vi "Billard2025.vi"(5 "Open pdf":bool=TRUE, 7 "ball size":i32=13, 8 "band touch win":u32(colorbox)=16711680, 9 "band touch loose":u32(colorbox)=6618880, 10 "Open Scoresheet":bool=TRUE, 11 "path to PNG file":path=path "/Users/leonkesselring/Desktop/LabView/Proj Prog/T1-2") -> (0 "error out":errorcluster={"status"=TRUE, "code"=-1, "source"="Script error. \n{\bError: File: /Users/leonkesselring/Desktop/LabView/Proj Prog/AnalyseT5.m Line:\n310 Column: 34\nThe function \"GetTouchIdx\" was closed with an 'end', but at least one other\nfunction definition was not. All functions in a script must be closed with an\n'end'.\n}\b \n"}, 1 "Summary output":string="Error -1 occurred at Script error. \n{\bError: File: /Users/leonkesselring/Desktop/LabView/Proj Prog/AnalyseT5.m Line:\n310 Column: 34\nThe function \"GetTouchIdx\" was closed with an 'end', but at least one other\nfunction definition was not. All functions in a script must be closed with an\n'end'.\n}\b\n\nThis error code is undefined. Undefined errors might occur for a number of reasons. For example, no one has provided a description for the code, or you might have wired a number that is not an error code to the error code input. \n\nAdditionally, undefined error codes might occur because the error relates to a third-party object, such as the operating system or ActiveX. For these third-party errors, you might be able to obtain a description of the error by searching the Web for the error code (-1) or for its hexadecimal representation (0xFFFFFFFF).")   [LabVIEW 2025]
panel:
  out "error out 3":errorcluster={"status"=TRUE, "code"=-1, "source"="Script error. \n{\bError: File: /Users/leonkesselring/Desktop/LabView/Proj Prog/AnalyseT5.m Line:\n310 Column: 34\nThe function \"GetTouchIdx\" was closed with an 'end', but at least one other\nfunction definition was not. All functions in a script must be closed with an\n'end'.\n}\b \n"}
  out "error out 2":errorcluster
  out "stripped path txt file 3":path=path "/Users/leonkesselring/Desktop/LabView/Proj Prog"
  out "name":string="T5"
  out "filenames":string[](array[string])=["1591.png", "1592.png", "1593.png", "1594.png", "1595.png", "1596.png", "1597.png", "1598.png", "1599.png", "1600.png", "1601.png", "1602.png", "1603.png", "1604.png", "1605.png", "1606.png", "1607.png", "1608.png", "1609.png", "1610.png", "1611.png", "1612.png", "1613.png", "1614.png", "1615.png", "1616.png", "1617.png", "1618.png", "1619.png", "1620.png", "1621.png", "1622.png", "1623.png", "1624.png", "1625.png", "1626.png", "1627.png", "1628.png", "1629.png", "1630.png", "1631.png", "1632.png", "1633.png", "1634.png", "1635.png", "1636.png", "1637.png", "1638.png", "1639.png", "1640.png", "1641.png", "1642.png", "1643.png", "1644.png", "1645.png", "1646.png", "1647.png", "1648.png", "1649.png", "1650.png", "1651.png", "1652.png", "1653.png", "1654.png", "1655.png", "1656.png", "1657.png", "1658.png", "1659.png", "1660.png", "1661.png", "1662.png", "1663.png", "1664.png", "1665.png", "1666.png", "1667.png", "1668.png", "1669.png", "1670.png", "1671.png", "1672.png", "1673.png", "1674.png", "1675.png", "1676.png", "1677.png", "1678.png", "1679.png", "1680.png", "1681.png", "1682.png", "1683.png", "1684.png", "1685.png", "1686.png", "1687.png", "1688.png", "1689.png", "1690.png", "1691.png", "1692.png", "1693.png", "1694.png", "1695.png", "1696.png", "1697.png", "1698.png", "1699.png", "1700.png", "1701.png", "1702.png", "1703.png", "1704.png", "1705.png", "1706.png", "1707.png", "1708.png", "1709.png", "1710.png", "1711.png", "1712.png", "1713.png", "1714.png", "1715.png", "1716.png", "1717.png", "1718.png", "1719.png", "1720.png", "1721.png", "1722.png", "1723.png", "1724.png", "1725.png", "1726.png", "1727.png", "1728.png", "1729.png", "1730.png", "1731.png", "1732.png"]
  out "String":string="T5"
  out "concatenated string":string="\n \nTlist;%% integrating \"InterpolateNan\" and \"RemoveOutlier\"\n\n% Interpolate missing values in the traces\n[Xr, Yr] = InterpolateNan(Xr, Yr);\n[Xy, Yy] = InterpolateNan(Xy, Yy);\n[Xw, Yw] = InterpolateNan(Xw, Yw);\n\n% Remove outliers from the traces\n[Xr, Yr] = RemoveOutlier(Xr, Yr);\n[Xy, Yy] = RemoveOutlier(Xy, Yy);\n[Xw, Yw] = RemoveOutlier(Xw, Yw);\n\n%% invert\nH = 480;\nYr = H - Yr;\nYy = H - Yy;\nYw = H - Yw;\n\n%% integrating \"GetFramme\"\n\n[Xmin, Xmax, Ymin, Ymax] = GetFrame(Xr, Yr, Xy, Yy, Xw, Yw);\n\n\n%% creat trace for frame\n\nxf = [Xmin Xmax Xmax Xmin Xmin];\nyf = [Ymin Ymin Ymax Ymax Ymin];\n\n%% integrating \"GetBallPathLength\" and \"GetFirstMoveIdx\"\nMoveDistPx = 9;\nLr = GetBallPathLength(Xr, Yr);\nLy = GetBallPathLength(Xy, Yy);\nLw = GetBallPathLength(Xw, Yw);\n\n[idxFirstR, DistMoveR] = GetFirstMoveIdx(Xr, Yr, MoveDistPx);\n[idxFirstY, DistMoveY] = GetFirstMoveIdx(Xy, Yy, MoveDistPx);\n[idxFirstW, DistMoveW] = GetFirstMoveIdx(Xw, Yw, MoveDistPx);\n\n%% integrating \"GetTouchIdx\" and \"GetBallMoveOrder\"\n\nBallBorderDist = 9;\nIdxTouchR = GetTouchIdx(Xr, Yr, Xmin, Xmax, Ymin, Ymax, BallBorderDist);\nIdxTouchY = GetTouchIdx(Xy, Yy, Xmin, Xmax, Ymin, Ymax, BallBorderDist);\nIdxTouchW = GetTouchIdx(Xw, Yw, Xmin, Xmax, Ymin, Ymax, BallBorderDist);\n\n[FirstBall, SecondBall, LastBall, NbBallsMoved] = GetBallMoveOrder(Xr, Yr, Xy, Yy, Xw, Yw, MoveDistPx);\n\nif FirstBall == 1\n    Xfirst = Xr;\n    Yfirst = Yr;\n    IdxTouchfirst = IdxTouchR;\n    ColorScore = 'red';\nelseif FirstBall == 2\n    Xfirst = Xy;\n    Yfirst = Yy;\n    IdxTouchfirst = IdxTouchY;\n    ColorScore = 'yellow';\nelse \n    Xfirst = Xw;\n    Yfirst = Yw;\n    IdxTouchfirst = IdxTouchW;\n    ColorScore = 'white';\nend\n\n%% determin Win/lose\n\nScore = GetWinnerScore(idxFirstR, idxFirstY, idxFirstW, IdxTouchfirst, NbBallsMoved);\n\nif strcmp(Score, 'win')\n    \n\ncolortouches = [1 0 0];\nelse\ncolortouches = [0 1 0];\nend\n%% Display the frame and traces\n\nfig = figure('Color','k'); % dark background\nax = axes(fig);\nset(ax,'Color','k'); \nhold(ax,'on'); \n\n% Frame in gray\nplot(ax, xf, yf, '-', 'LineWidth', 1.5, 'Color', [0.6 0.6 0.6]);\n\n% Traces: R, Y, W\nplot(ax, Xr, Yr, 'o-', 'LineWidth', 1.6, 'Color', [1 0 0]);   % red\nplot(ax, Xy, Yy, 'o-', 'LineWidth', 1.6, 'Color', [1 1 0]);   % yellow\nplot(ax, Xw, Yw, 'o-', 'LineWidth', 1.6, 'Color', 'b');       % white ball (blue trace)\n\n% Plot touches for first ball\nplot(ax, Xfirst(IdxTouchfirst), Yfirst(IdxTouchfirst), 'o', ...\n     'MarkerSize', 30, 'Color', colortouches);\n\n% Plot origins\nplot(ax, Xr(1), Yr(1), 'hexagram', 'MarkerSize', 20, 'Color', [1 0 0]);\nplot(ax, Xy(1), Yy(1), 'hexagram', 'MarkerSize', 20, 'Color', [1 1 0]);\nplot(ax, Xw(1), Yw(1), 'hexagram', 'MarkerSize', 20, 'Color', 'b');\n\n% Design: frame sizing\naxis(ax,'equal');\naxis(ax,[Xmin Xmax Ymin Ymax]);\n\naxis(ax,'off');   \n\ntitle(ax, ['Scores sheet -T5 - ' datestr(now,'yyyy-mm-dd - HH:MM')], ...\n    'Color', 'w', 'FontSize', 14);\n\n\n%% Legend area below the frame\n\npadBottom = 0.20*(Ymax - Ymin);   \naxis(ax,[Xmin Xmax Ymin - padBottom Ymax]);\n\nxl = xlim(ax);\nyl = ylim(ax);\n\nxLeft   = xl(1) + 0.05*(xl(2)-xl(1));\nxCenter = xl(1) + 0.40*(xl(2)-xl(1));\nxRight  = xl(1) + 0.80*(xl(2)-xl(1));\nyBase   = yl(1) + 0.15*(Ymax - Ymin);\n\nNbBandsTouched = numel(IdxTouchfirst);\n\n% Winner section\nV = [idxFirstR idxFirstY idxFirstW];\nVsort = sort(V);\n\nif NbBallsMoved == 3   % only then Vsort has 3 elements\n    count = IdxTouchfirst( (Vsort(2) < IdxTouchfirst) & (IdxTouchfirst < Vsort(3)) );\n    NbBandsWin = numel(count);\nelse\n    NbBandsWin = 0;\nend\n\nif NbBallsMoved == 3 && NbBandsWin >= 3\n    Score = 'win';\nelse\n    Score = 'lose';\nend\n\n\ntext(xLeft, yBase, sprintf('Score sheet for \"%s\"', ColorScore), 'Color', 'w', 'FontSize', 12);\ntext(xLeft, yBase-30, sprintf('--- %s ---', Score), 'Color', 'w', 'FontSize', 12);\n\n% Distances\ntext(xLeft,   yBase-80, sprintf('red_d : %.0fpx',   Lr), 'Color', 'w', 'FontSize', 12);\ntext(xCenter, yBase-80, sprintf('yellow_d : %.0fpx', Ly), 'Color', 'w', 'FontSize', 12);\ntext(xRight,  yBase-80, sprintf('white_d : %.0fpx', Lw), 'Color', 'w', 'FontSize', 12);\n\n% Ball & band stats\ntext(xRight, yBase,   sprintf('%d ball(s) moved',   NbBallsMoved),   'Color', 'w', 'FontSize', 12);\ntext(xRight, yBase-30, sprintf('%d band(s) touched', NbBandsTouched), 'Color', 'w', 'FontSize', 12);\n\n%% PDF\nSeqName = 'T5';   % or pass this as a variable instead of hardcoding\r\n\r\npdfName = sprintf('ScoreSheet%s.pdf', SeqName);\r\nexportgraphics(fig, pdfName, 'ContentType','vector');\r\n\r\n%% Summary\r\n\r\n% Map ColorScore to char: f:[w,y,r]\r\nswitch lower(ColorScore)\r\n    case 'white'\r\n        fChar = 'w';\r\n    case 'yellow'\r\n        fChar = 'y';\r\n    case 'red'\r\n        fChar = 'r';\r\n    otherwise\r\n        fChar = 'x';   % unknown, for safety\r\nend\r\n\r\n% Map Score 'win'/'lose' to s:[w,l]\r\nif strcmpi(Score, 'win')\r\n    sChar = 'w';\r\nelse\r\n    sChar = 'l';\r\nend\r\n\r\n% Round distances to integers\r\nrb = round(Lr);\r\nyb = round(Ly);\r\nwb = round(Lw);\r\n\r\nsummaryStr = sprintf('f:%c; s:%c; n:%d; b:%d; rb:%d; yb:%d; wb:%d;', ...\r\n    fChar, sChar, NbBallsMoved, NbBandsTouched, rb, yb, wb);\r\n\r\nSummaryName = sprintf('Summary%s.txt', SeqName);\r\n\r\nfid = fopen(SummaryName, 'w');\r\nfprintf(fid, '%s\\n', summaryStr);\r\nfclose(fid);\r\n\r\n%% function InterpolateNan\r\n\r\nfunction [X, Y] = InterpolateNan(X, Y)\r\n\r\n    if isnan(X(1)),  X(1)  = 0; end\r\n    if isnan(X(end)),X(end)= 0; end\r\n\r\n    defX = ~isnan(X);\r\n    idX = 1:numel(X);\r\n    idx_defX = find(defX);\r\n    X =interp1(idx_defX,X(defX),idX,'next');\r\n\r\n    if isnan(Y(1)),  Y(1)  = 0; end\r\n    if isnan(Y(end)),Y(end)= 0; end\r\n\r\n    defY = ~isnan(Y);\r\n    idY = 1:numel(Y);\r\n    idx_defY = find(defY);\r\n    Y =interp1(idx_defY,Y(defY),idY,'next');\r\nend\r\n%% function RemoveOutlier\r\n\r\nfunction [X, Y] = RemoveOutlier(X, Y)\r\n    OX =isoutlier(X,'movmedian',10);\r\n    OY =isoutlier(Y,'movmedian',10);\r\n\r\n    O = OX & OY;\r\n    idx = find(O);\r\n    idx = idx(idx > 1);\r\n    \r\n    X(idx) = X(idx - 1);\r\n    Y(idx) = Y(idx - 1);\r\nend\r\n\r\n%% function GetFrame\r\n\r\nfunction [Xmin, Xmax, Ymin, Ymax] = GetFrame(Xr, Yr, Xy, Yy, Xw, Yw)\r\n    Xmin = min([Xr(:); Xy(:); Xw(:)], [], 'omitnan');\r\n    Xmax = max([Xr(:); Xy(:); Xw(:)], [], 'omitnan');\r\n    Ymin = min([Yr(:); Yy(:); Yw(:)], [], 'omitnan');\r\n    Ymax = max([Yr(:); Yy(:); Yw(:)], [], 'omitnan');\r\nend\r\n\r\n%% function GetBallPathLenght\r\n\r\nfunction PathLength = GetBallPathLength(X, Y)\r\n    dx = diff(X); \r\n    dy = diff(Y);\r\n    PathLength = sum( sqrt(dx.^2 + dy.^2) );\r\nend\r\n\r\n%% function GetFirstMoveIdx\r\n\r\nfunction [FirstMoveIdx, MoveDist] = GetFirstMoveIdx(X, Y, MoveDistPx)\r\n\r\n    X = X(:); \r\n    Y = Y(:);\r\n\r\n    % 1) Distances per segment \r\n    MoveDist = hypot(diff(X), diff(Y));     % length = N-1\r\n\r\n    % 2) Distance from initial position \r\n    DistFromStart = hypot(X - X(1), Y - Y(1));  % length = N\r\n\r\n    FirstMoveIdx = find(DistFromStart > MoveDistPx, 1, 'first');\r\n    if isempty(FirstMoveIdx)\r\n        FirstMoveIdx = [];  % as required: return [] if never moved\r\n    end\r\nend\r\n\r\n\r\n%% function GetTouchIdx\r\n\r\nfunction IdxTouch = GetTouchIdx(X, Y, Xmin, Xmax, Ymin, Ymax, BallBorderDist)\r\n%GETTOUCHIDX  Return time indices where the ball first touches a cushion.\r\n% A \"touch\" happens when the ball is closer than BallBorderDist to any\r\n% table border. Only the *first* index of each consecutive run is kept.\r\n\r\n    if nargin < 7 || isempty(BallBorderDist)      \nBallBorderDist = 9;            \r\n    end\r\n\r\n    % Ensure column vectors\r\n    X = X(:);  Y = Y(:);\r\n\r\n    % Logical masks: near each border\r\n    nearLeft   = (X - Xmin) < BallBorderDist;\r\n    nearRight  = (Xmax - X) < BallBorderDist;\r\n    nearBottom = (Y - Ymin) < BallBorderDist;\r\n    nearTop    = (Ymax - Y) < BallBorderDist;\r\n\r\n    % Helper: first index of every 0->1 transition (start of a \"touch\" run)\r\n    firstRunIdx = @(m) find(diff([false; m(:)]) == 1);\r\n\r\n    % Indices per border\r\n    idxL = firstRunIdx(nearLeft);\r\n    idxR = firstRunIdx(nearRight);\r\n    idxB = firstRunIdx(nearBottom);\r\n    idxT = firstRunIdx(nearTop);\r\n\r\n    % Merge borders, sort, deduplicate\r\n    IdxTouch = unique([idxL; idxR; idxB; idxT]);\r\n\r\n    % Omit index 1 if present (spec requirement)\r\n    IdxTouch(IdxTouch == 1) = [];\r\n\r\n    % If nothing touched, IdxTouch will naturally be []\r\nend\r\n\r\n%% function GetBallMoveOrder\n\nfunction [FirstBall, SecondBall, LastBall, NbBallsMoved] = ...\n    GetBallMoveOrder(Xr, Yr, Xy, Yy, Xw, Yw, MoveDistPx)\n%GETBALLMOVEORDER  Determine which ball moves first, second, and third.\n% Balls: Red=1, Yellow=2, White=3.\n%\n% Ranking rules:\n%   1) Primary key  : earliest FirstMoveIdx\n%   2) Tie-breaker  : larger first segment distance (MoveDist(1))\n%   3) Non-movers   : get index length(X)+1 (sorted to the end)\n%\n% Outputs:\n%   FirstBall, SecondBall, LastBall : labels 1/2/3\n%   NbBallsMoved : number of balls that actually moved\n\n    % --- Gather features for each ball (idx, firstSeg, len) ---\n    [idxR, segR, nR] = FirstMoveFeatures_NoNest(Xr, Yr, MoveDistPx); % Red   -> 1\n    [idxY, segY, nY] = FirstMoveFeatures_NoNest(Xy, Yy, MoveDistPx); % Yellow-> 2\n    [idxW, segW, nW] = FirstMoveFeatures_NoNest(Xw, Yw, MoveDistPx); % White -> 3\n\n    ids   = [1;      2;      3     ];\n    idxs  = [idxR;   idxY;   idxW  ];\n    segs  = [segR;   segY;   segW  ];\n    lens  = [nR;     nY;     nW    ];\n\n    % Count movers (idx <= actual length of that ball's track)\n    NbBallsMoved = sum(idxs <= lens);\n\n    % Sort by (idx ascending, firstSeg descending)\n    sortMat = [idxs, -segs];\n    [~, order] = sortrows(sortMat, [1 2]);\n\n    orderedIds = ids(order);\n\n    FirstBall  = orderedIds(1);\n    SecondBall = orderedIds(2);\n    LastBall   = orderedIds(3);\nend\n\n%% helper for GetBallMoveOrder (NOT nested)\n\nfunction [idx, firstSeg, n] = FirstMoveFeatures_NoNest(X, Y, MoveDistPx)\n%FIRSTMOVEFEATURES_NONEST Return (firstMoveIdx, firstSegmentDistance, trackLength)\n% Non-movers are assigned idx = n+1 so they sort last.\n\n    n = numel(X);\n\n    [idxFound, moveDist] = GetFirstMoveIdx(X, Y, MoveDistPx);\n\n    % Non-mover handling\n    if isempty(idxFound) || ~isfinite(idxFound) || idxFound < 1\n        idx = n + 1;   % treated as non-mover\n    else\n        idx = idxFound;\n    end\n\n    % Tie-breaker: first segment distance\n    if isempty(moveDist)\n        firstSeg = 0;\n    else\n        firstSeg = moveDist(1);\n    end\nend\n\r\n%% Winner function\r\n\r\nfunction Score = GetWinnerScore(idxFirstR, idxFirstY, idxFirstW, IdxTouchfirst, NbBallsMoved)\r\n    V = [idxFirstR idxFirstY idxFirstW];\r\n    Vsort = sort(V);\r\n    \r\n    if NbBallsMoved == 3   % only then Vsort has 3 elements\r\n        count = IdxTouchfirst(( Vsort(2) < IdxTouchfirst) & (IdxTouchfirst < Vsort(3)) );\r\n        NbBandsWin = numel(count);\r\n    else\r\n        NbBandsWin = 0;\r\n    end\r\n    \r\n    if NbBallsMoved == 3 && NbBandsWin >= 3\r\n        Score = 'win';\r\n    else\r\n        Score = 'lose';\r\n    end\r\nend\n"
  in  "Create PDF":bool=TRUE
  in  "Count Summary":i32=-1
  out "computed command line":string="[\bWarning: Command line argument -sd has already been specified.\n-useStartupFolderPref will be ignored.]\b \n"
  out "White Last":i32=121
  out "Yellow Last":i32=87
  out "Red Last":i32=120
  in  "RGB Values Border":T1={"Border Rmin"=0.0, "Border Rmax "=24.0, "Border Gmin "=0.0, "Border Gmax"=49.0, "Border Bmin"=100.0, "Border Bmax"=119.0}
  out "offset past scan":u32=60
  out "RGB Values Background 2":T2={"BG Blue Rmin"=46.0, "BG Blue Rmax "=63.0, " BG Blue Gmin"=93.0, "BG Blue Gmax"=150.0, "BG Blue Bmin "=150.0, "Bg Blue Bmax"=185.0}
  in  "wait until completion? (T)":bool=TRUE
  out "stripped path txt file 2":path=path "/Users/leonkesselring/Desktop/LabView/Proj Prog"
  out "RGB Values Balls":string="91 255 0 80 0 130 170 255 176 255 0 175 100 255 150 255 150 255"
  in  "RGB Values Background":T2={"BG Blue Rmin"=46.0, "BG Blue Rmax "=63.0, " BG Blue Gmin"=93.0, "BG Blue Gmax"=150.0, "BG Blue Bmin "=150.0, "Bg Blue Bmax"=185.0}
  in  "RGB Values Balls":T3={"BRed Rmin"=91, "BRed Rmax"=255, "BRed Gmin"=0, "BYel Rmin"=170, "BYel Rmax"=255, " BYel Gmin"=176, "BRed Gmax"=80, "BYel Gmax "=255, "BRed Bmin"=0, "BYel Bmin"=0, "BRed Bmax"=130, " BYel Bmax"=175, "BWhite Rmin"=100, "BWhite Rmax"=255, "BWhite Gmin"=150, "BWhite Gmax"=255, "BWhite Bmin"=150, "BWhite Bmax"=255}
  out "T list string":string="Xr=[230 230 230 230 230 230 230 230 230 230 230 230 230 230 230 230 230 230 230 230 230 230 230 230 230 230 230 230 230 230 230 230 230 230 230 230 230 230 230 230 230 230 230 230 230 230 230 230 230 230 230 230 230 230 230 230 230 230 230 230 230 230 230 230 230 230 230 230 230 230 225 221 213 210 206 203 195 192 189 185 179 175 172 168 162 158 155 151 145 142 139 136 129 128 131 131 136 137 139 140 144 145 147 149 151 153 155 156 159 161 163 164 167 168 170 172 175 176 178 179 182 183 184 186 189 190 191 193 195 196 198 199 201 202 203 205 207 209 209 211 213 213 ];Yr=[319 319 319 319 319 319 319 319 319 319 319 319 319 319 319 319 319 319 319 319 319 319 319 319 319 319 319 319 319 319 319 319 319 319 319 319 319 319 319 319 319 319 319 319 319 319 319 319 319 319 319 319 319 319 319 319 319 319 319 319 319 319 319 319 319 319 319 319 319 319 315 312 306 303 301 297 291 290 287 285 280 277 274 271 267 264 261 259 255 252 249 247 242 239 239 237 233 231 229 229 225 223 222 221 217 216 214 213 210 209 207 206 203 202 200 198 195 194 193 191 189 187 187 185 183 181 180 179 176 175 174 173 171 169 168 167 165 163 163 161 159 159 ];Xy=[243 243 243 243 243 243 243 243 243 243 243 243 243 243 243 243 243 243 243 243 243 243 243 243 243 243 243 243 243 243 243 243 243 243 243 243 243 243 243 243 243 243 243 243 243 243 243 243 243 243 243 243 243 243 243 243 243 243 243 243 243 243 243 243 243 243 243 243 243 243 243 243 243 243 243 243 243 243 243 243 243 243 243 243 243 243 243 243 243 243 243 243 243 243 243 243 243 243 243 243 243 243 243 243 243 243 243 243 243 243 243 243 243 243 243 243 243 243 243 243 243 243 243 243 243 243 243 243 243 243 243 243 242 242 242 242 242 242 242 242 242 242 ];Yy=[344 344 344 344 344 344 344 344 344 344 344 344 344 344 344 344 344 344 344 344 344 344 344 344 344 344 344 344 344 344 344 344 344 344 344 344 344 344 344 344 344 344 344 344 344 344 344 344 344 344 344 344 344 344 344 344 344 344 344 344 344 344 344 344 344 344 344 344 344 344 344 344 344 344 344 344 344 344 344 344 344 344 344 344 344 344 344 344 344 344 344 344 344 344 344 344 344 344 344 344 344 344 344 344 344 344 344 344 344 344 344 344 344 344 344 344 344 344 344 344 344 344 344 344 344 344 344 344 344 344 344 344 344 344 344 344 344 344 344 344 344 344 ];Xw=[239 239 239 239 245 265 284 302 340 359 378 397 434 453 472 491 527 545 563 580 616 635 652 670 705 723 720 705 676 663 651 641 621 612 603 595 578 569 560 552 535 526 518 509 492 484 476 467 451 442 434 426 409 401 393 385 368 360 352 344 328 320 312 304 288 280 272 264 248 241 237 234 227 223 219 215 208 204 200 197 189 186 182 178 171 167 164 160 153 149 146 143 136 132 129 128 133 135 137 138 142 144 146 147 151 152 154 156 159 161 162 164 167 168 169 171 173 175 176 178 180 181 182 184 186 187 188 190 192 193 194 195 197 198 199 200 202 203 204 205 207 208 ];Yw=[368 368 368 368 369 370 372 373 377 380 382 383 387 389 391 392 391 390 389 387 386 385 384 383 381 380 382 385 390 392 391 389 386 384 383 382 379 378 376 375 373 371 370 369 367 365 364 362 360 359 357 356 354 352 351 350 347 346 345 343 341 339 338 337 335 333 332 331 328 327 329 332 336 337 339 341 344 346 348 350 353 355 356 358 361 363 365 366 369 371 373 374 378 379 381 382 383 383 384 385 386 387 388 388 390 390 391 391 392 393 393 393 393 393 393 392 391 391 391 390 390 390 389 389 388 388 388 387 387 386 386 386 386 385 385 385 384 384 384 383 383 383 ];"
  out "stripped path txt file":path=path "/Users/leonkesselring/Desktop/LabView/Proj Prog"
  out "Y White":i32=383
  out "X White":i32=208
  out "Y Yellow":i32=344
  out "X Yellow":i32=242
  out "Y Red":i32=159
  out "X Red":i32=213
  out "Bornes":T4={"Xmin"=127, "Xmax"=739, "Ymin"=101, "Ymax"=406}
  in  "run minimized? (F)":bool
  out "C part standard error":string
  out "C part standard output":string
  in  "count":i32=-1
  out "text":string="Red: 213, 159, 120\nYellow: 242, 344, 87\nWhite: 208, 383, 121\n"
  out "Stripped path for pixmap.bin":path=path "/Users/leonkesselring/Desktop/LabView/Proj Prog"
  out "Pixmap.bin":u32[](array[numeric])
  out "24-bit pixmap":u32[][](array[numeric]) format="%x"
  out "hauteur":i16=480
  out "largeur":i16=854
  out "image":u8[](array[numeric])
  out "Image depth":i32=24
  out "PNG Picture":picture
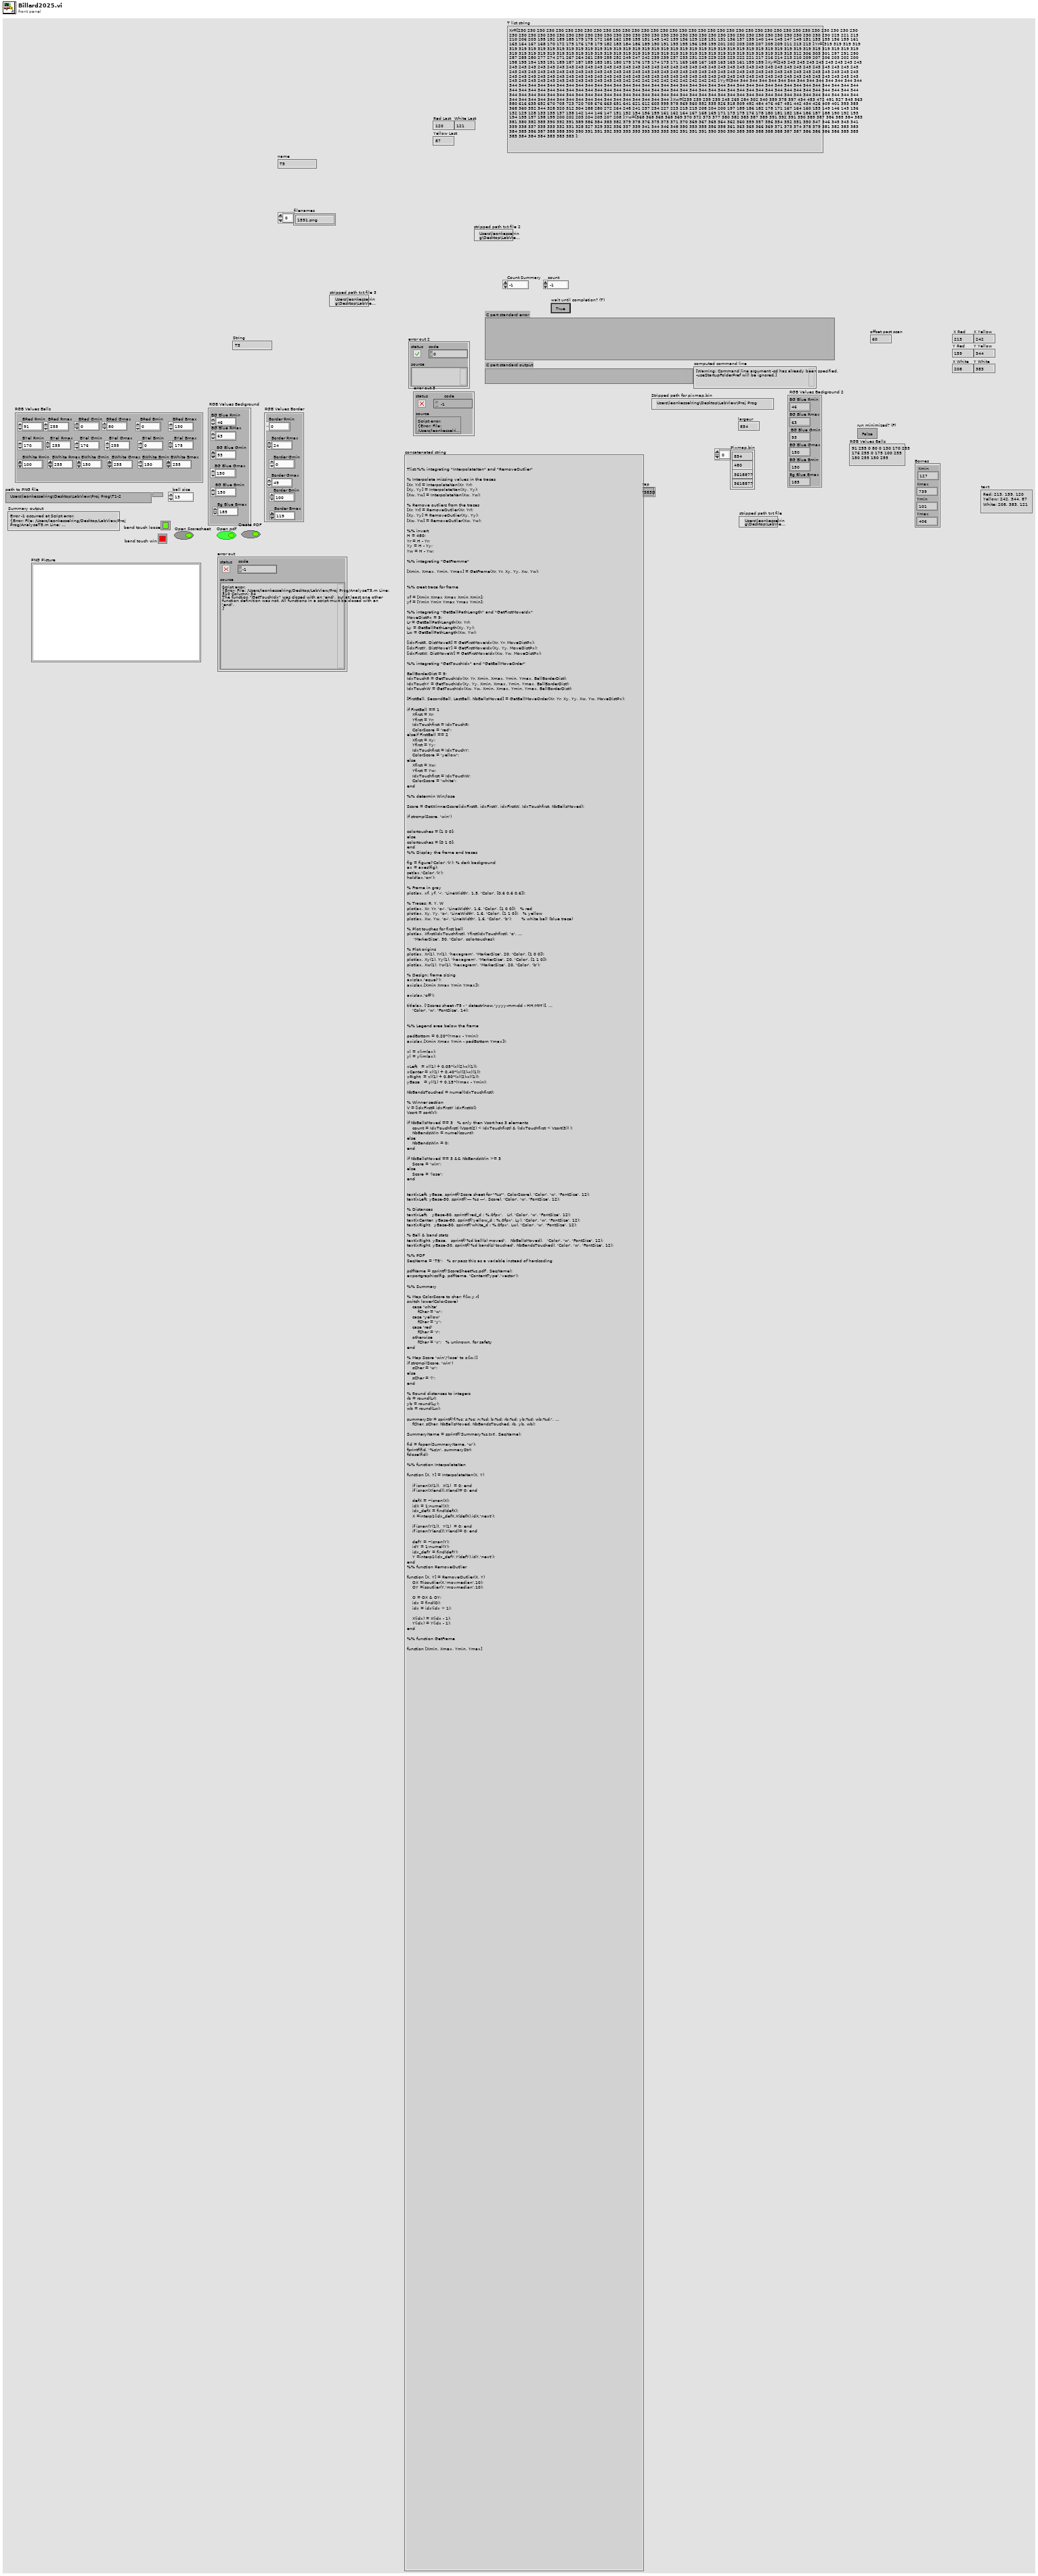
[diagram p1: front panel]
types:
  T1 = cluster{"Border Rmin":dbl, "Border Rmax ":dbl, "Border Gmin ":dbl, "Border Gmax":dbl, "Border Bmin":dbl, "Border Bmax":dbl}
  T2 = cluster{"BG Blue Rmin":dbl, "BG Blue Rmax ":dbl, " BG Blue Gmin":dbl, "BG Blue Gmax":dbl, "BG Blue Bmin ":dbl, "Bg Blue Bmax":dbl}
  T3 = cluster{"BRed Rmin":i32, "BRed Rmax":i32, "BRed Gmin":i32, "BYel Rmin":i32, "BYel Rmax":i32, " BYel Gmin":i32, "BRed Gmax":i32, "BYel Gmax ":i32, "BRed Bmin":i32, "BYel Bmin":i32, "BRed Bmax":i32, " BYel Bmax":i32, "BWhite Rmin":i32, "BWhite Rmax":i32, "BWhite Gmin":i32, "BWhite Gmax":i32, "BWhite Bmin":i32, "BWhite Bmax":i32}
  T4 = cluster{"Xmin":i32, "Xmax":i32, "Ymin":i32, "Ymax":i32}
  T5 = enum16{"big-endian, network order", "native, host order", "little-endian"}
  T6 = enum16{"open", "replace", "create", "open or create", "replace or create", "replace or create with confirmation"}
  T7 = typedef "imagedata.ctl" = cluster{"image type":i32, "image depth":i32, "image":u8[], "mask":u8[], "colors":u32[], "Rectangle":cluster{"left":i16, "top":i16, "right":i16, "bottom":i16}}
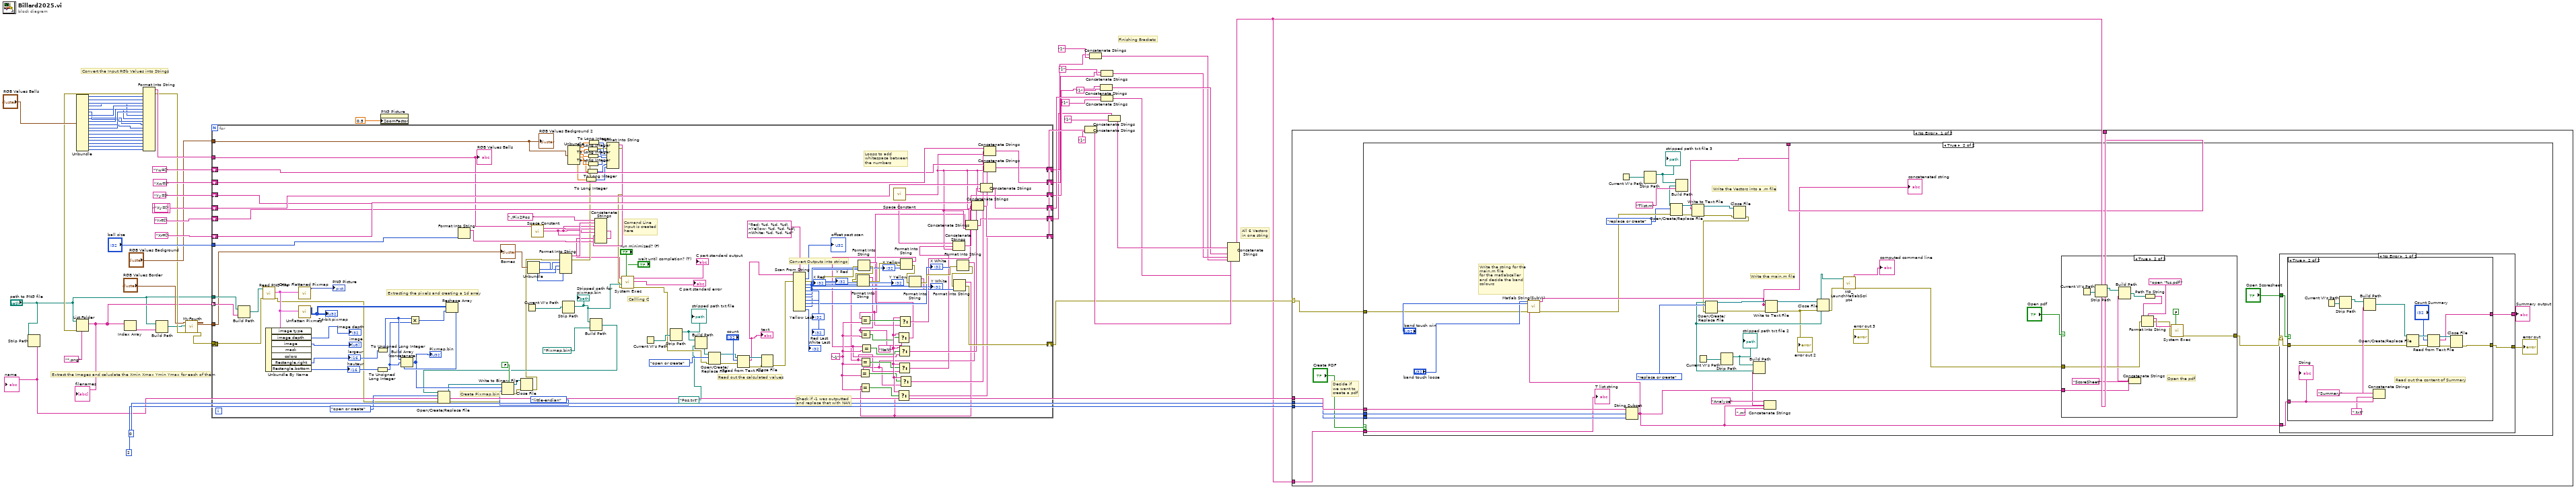
[diagram p0: block diagram]
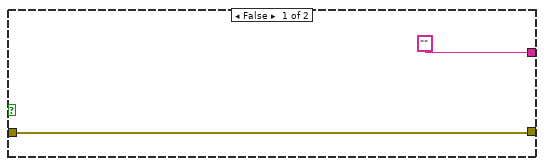
[diagram p3: hidden frame]
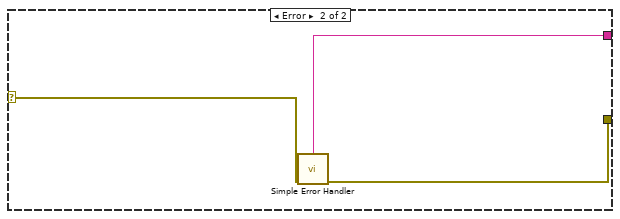
[diagram p4: hidden frame]
diagram:
  (unwired) "Xy=["
  # "All 6 Vectors\nin one string"
  # "Finishing Brackets"
  # "Extract the Images and caluclate the Xmin Xmax Ymin Ymax for each of them"
  # "Convert the Input RGb Values into Strings"
  n1 = Strip Path(path="path to PNG file") -> (name=w3:string)  [unwired: 1 out]
  "name" <- w3
  n2 = Unbundle("RGB Values Balls") -> ("BRed Rmin"=w30:i32, "BRed Rmax"=w29:i32, "BRed Gmin"=w27:i32, "BYel Rmin"=w23:i32, "BYel Rmax"=w22:i32, "BYel Gmin"=w21:i32, "BRed Gmax"=w26:i32, "BYel Gmax"=w20:i32, "BRed Bmin"=w25:i32, "BYel Bmin"=w19:i32, "BRed Bmax"=w24:i32, "BYel Bmax"=w18:i32, "BWhite Rmin"=w17:i32, "BWhite Rmax"=w16:i32, "BWhite Gmin"=w15:i32, "BWhite Gmax"=w14:i32, "BWhite Bmin"=w13:i32, "BWhite Bmax"=w12:i32)
  n3 = List Folder(path="path to PNG file", pattern="*.png") -> (filenames=w6:string[], error out=w28:errorcluster)  [unwired: 2 in, 2 out]
  "filenames" <- w6
  n4 = Index Array(array=w6) -> (element=w4:string)  [unwired: 1 in]
  n5 = Format Into String(error in=w28, w30, w29, w27, w26, w25, w24, w23, w22, w21, w20, w19, w18, w17, w16, w15, w14, w13, w12) -> (resulting string=w36:string, error out=w9:errorcluster)  [unwired: 2 in]
  n6 = Build Path(base path="path to PNG file", name or relative path=w4) -> (appended path=w7:path)
  n7 = call "MyFourth.vi"("error in (no error)"=w9, "path to JPEG file"=w7, "Border"="RGB Values Border") -> ("error out"=w8:errorcluster, "Bornes"=w10:cluster{i32, i32, "Ymin":i32, "Ymax":i32})  [unwired: 7 in]
  n8 = for {
    tunnel: "path to PNG file" -> [w174]
    tunnel: w6 -> [w175] mode=indexing
    tunnel: w10 -> [w141]
    tunnel: w8 -> [w172]
    shift-right: [w152] -> w60
    shift-left: "Xr=[" -> [w154]
    shift-right: [w146] -> w2
    shift-left: "Yr=[" -> [w151]
    shift-right: [w145] -> w48
    shift-left: "Xy=[" -> [w150]
    shift-right: [w144] -> w47
    shift-left: "Yy=[" -> [w149]
    shift-right: [w143] -> w46
    shift-left: "Xw=[" -> [w148]
    shift-right: [w142] -> w45
    shift-left: "Yw=[" -> [w147]
    tunnel: "ball size" -> [w138]
    tunnel: w36 -> [w133]
    shift-right: [w95] -> w31
    shift-left: _ -> [_]
    tunnel: "RGB Values Background" -> [w132]
    w81 = "-1"
    w80 = "NaN"
    # "Read out the calculated values"
    # "Callling C"
    # "Extracting the pixels and creating a 1d array"
    # "Loops to add\nwhitespace between\nthe numbers"
    # "Convert Outputs into strings"
    # "Check if -1 was outputted\nand replace that with NAN"
    # "Create Pixmap.bin"
    # "Comand Line\nInput is created\nhere"
    n9 = Build Path(base path=w174, name or relative path=w175) -> (appended path=w173:path)
    n10 = call <vilib>:"Read PNG File.vi"("error in (no error)"=w172, "path to PNG file"=w173) -> ("error out"=w111:errorcluster, "image data"=w184:T7)  [unwired: 7 in, 1 out]
    n11 = Unbundle By Name(w184) -> ("image depth"=→"Image depth":i32, "image"=→"image":u8[], "Rectangle.right"=w181:i16, "Rectangle.bottom"=w179:i16)  [unwired: 3 out]
    "largeur" <- w181
    "hauteur" <- w179
    n12 = call <vilib>:"Draw Flattened Pixmap.vi"("image data"=w184) -> ("new picture"=→"PNG Picture":picture)  [unwired: 8 in]
    n13 = call <vilib>:"Unflatten Pixmap.vi"("image data"=w184) -> ("24-bit pixmap"=w183:u32[][])  [unwired: 4 in, 6 out]
    "24-bit pixmap" <- w183
    n14 = To Unsigned Long Integer(number=w179) -> (unsigned 32bit integer=w178:u32)
    n15 = To Unsigned Long Integer(number=w181) -> (unsigned 32bit integer=w180:u32)
    n16 = Multiply(x=w180, y=w178) -> (x*y=w177:u32)
    n17 = Reshape Array(w183, w177) -> (w182:u32[])
    n18 = Build Array (concatenate)(w180, w178, w182) -> (w176:u32[])
    "Pixmap.bin" <- w176
    n19 = Format Into String(w138) -> (resulting string=w129:string)  [unwired: 3 in, 1 out]
    n20 = Current VI's Path() -> (path=w163:path)
    n21 = Unbundle(w141) -> (w114:i32, w113:i32, "Ymin"=w116:i32, "Ymax"=w115:i32)
    n22 = call <vilib>:"Space Constant.vi"() -> ("String"=w130:string)
    n23 = Strip Path(path=w163) -> (stripped path=w134:path)  [unwired: 1 out]
    "Stripped path for pixmap.bin" <- w134
    n24 = Unbundle(w132) -> ("BG Blue Rmin"=w128:dbl, "BG Blue Rmax"=w126:dbl, "BG Blue Gmin"=w124:dbl, "BG Blue Gmax"=w122:dbl, "BG Blue Bmin"=w120:dbl, "Bg Blue Bmax"=w118:dbl)
    n25 = To Long Integer(number=w118) -> (32bit integer=w117:i32)
    n26 = To Long Integer(number=w120) -> (32bit integer=w119:i32)
    n27 = To Long Integer(number=w126) -> (32bit integer=w125:i32)
    n28 = To Long Integer(number=w124) -> (32bit integer=w123:i32)
    n29 = To Long Integer(number=w122) -> (32bit integer=w121:i32)
    n30 = To Long Integer(number=w128) -> (32bit integer=w127:i32)
    n31 = Build Path(base path=w134, name or relative path=path "Pixmap.bin") -> (appended path=w158:path)
    n32 = Open/Create/Replace File(file path (use dialog)=w158, error in=w111, operation (0:open)=T6."open or create") -> (refnum out=w171:refnum<file>, error out=w110:errorcluster)  [unwired: 3 in, 1 out]
    n33 = Write to Binary File(file (use dialog)=w171, data=w176, error in=w110, 5:FALSE ("prepend array or string size? (T)"), 9:T5."little-endian" ("byte order (0:big-endian, network order)")) -> (refnum out=w160:refnum<file>, error out=w109:errorcluster)  [unwired: 1 in, 1 out]
    n34 = Close File(refnum=w160, error in=w109) -> (error out=w104:errorcluster)  [unwired: 1 out]
    n35 = Format Into String(error in=w104, w116, w115, w114, w113) -> (resulting string=w139:string, error out=w103:errorcluster)  [unwired: 2 in]
    n36 = Format Into String(error in=w103, w127, w125, w123, w121, w119, w117) -> (resulting string=w131:string, error out=w102:errorcluster)  [unwired: 2 in]
    n37 = Concatenate Strings("./Pix2Pos  ", w139, w130, w133, w130, w131, w130, w129) -> (w84:string)
    n38 = call <vilib>:"System Exec.vi"("run minimized? (F)"="run minimized? (F)", "wait until completion? (T)"="wait until completion? (T)", "error in (no error)"=w102, "working directory"=w134, "command line"=w84) -> ("error out"=w108:errorcluster, "standard error"=→"C part standard error":string, "standard output"=→"C part standard output":string)  [unwired: 3 in, 1 out]
    n39 = Current VI's Path() -> (path=w157:path)
    n40 = Strip Path(path=w157) -> (stripped path=w156:path)  [unwired: 1 out]
    "stripped path txt file" <- w156
    n41 = Build Path(base path=w156, name or relative path=path "Pos.txt") -> (appended path=w155:path)
    n42 = Open/Create/Replace File(file path (use dialog)=w155, error in=w108, operation (0:open)=T6."open or create") -> (refnum out=w164:refnum<file>, error out=w167:errorcluster)  [unwired: 3 in, 1 out]
    n43 = Read from Text File(file (use dialog)=w164, count="count", error in=w167) -> (refnum out=w165:refnum<file>, text=w93:string, error out=w168:errorcluster)  [unwired: 1 in, 1 out]
    "text" <- w93
    n44 = Close File(refnum=w165, error in=w168) -> (error out=w105:errorcluster)  [unwired: 1 out]
    n45 = Scan From String(format string="Red: %d, %d, %d\nYellow: %d, %d, %d\nWhite: %d, %d, %d", input string=w93, error in=w105) -> (offset past scan=→"offset past scan":u32, error out=w101:errorcluster, output 1=w82:i32, output 2=w153:i32, output 3=→"Red Last":i32, output 4=w90:i32, output 5=w89:i32, output 6=→"Yellow Last":i32, output 7=w87:i32, output 8=w86:i32, output 9=→"White Last":i32)  [unwired: 10 in, 1 out]
    "X Red" <- w82
    "Y Red" <- w153
    "X Yellow" <- w90
    "Y Yellow" <- w89
    "X White" <- w87
    "Y White" <- w86
    n46 = Format Into String(error in=w101, w82) -> (resulting string=w74:string, error out=w100:errorcluster)  [unwired: 2 in]
    n47 = Format Into String(error in=w100, w153) -> (resulting string=w72:string, error out=w99:errorcluster)  [unwired: 2 in]
    n48 = Equal?(x=w74, y=w81) -> (x = y?=w83:bool)
    n49 = Equal?(x=w72, y=w81) -> (x = y?=w79:bool)
    n50 = call <vilib>:"Space Constant.vi"() -> ("String"=w137:string)
    n51 = Select(t=w80, s=w79, f=w72) -> (s? t:f=w71:string)
    n52 = Select(t=w80, s=w83, f=w74) -> (s? t:f=w73:string)
    n53 = Format Into String(error in=w99, w90) -> (resulting string=w70:string, error out=w98:errorcluster)  [unwired: 2 in]
    n54 = Equal?(x=w70, y=w81) -> (x = y?=w78:bool)
    n55 = Select(t=w80, s=w78, f=w70) -> (s? t:f=w69:string)
    n56 = Format Into String(error in=w98, w89) -> (resulting string=w68:string, error out=w97:errorcluster)  [unwired: 2 in]
    n57 = Equal?(x=w68, y=w81) -> (x = y?=w77:bool)
    n58 = Select(t=w80, s=w77, f=w68) -> (s? t:f=w67:string)
    n59 = Concatenate Strings(w149, w67, w137) -> (w144:string)
    n60 = Format Into String(error in=w97, w87) -> (resulting string=w66:string, error out=w96:errorcluster)  [unwired: 2 in]
    n61 = Equal?(x=w66, y=w81) -> (x = y?=w76:bool)
    n62 = Select(t=w80, s=w76, f=w66) -> (s? t:f=w65:string)
    n63 = Format Into String(error in=w96, w86) -> (resulting string=w64:string, error out=w95:errorcluster)  [unwired: 2 in]
    n64 = Equal?(x=w64, y=w81) -> (x = y?=w75:bool)
    n65 = Select(t=w80, s=w75, f=w64) -> (s? t:f=w63:string)
    n66 = Concatenate Strings(w151, w71, w137) -> (w146:string)
    n67 = Concatenate Strings(w154, w73, w137) -> (w152:string)
    n68 = Concatenate Strings(w150, w69, w137) -> (w145:string)
    n69 = Concatenate Strings(w148, w65, w137) -> (w143:string)
    n70 = Concatenate Strings(w147, w63, w137) -> (w142:string)
    "Bornes" <- w141
    "RGB Values Balls" <- w133
    "RGB Values Background 2" <- w132
  }
  n71 = property on="PNG Picture" class="Pict"("ZoomFactor"=sgl 0.5 ("Zoom Factor")) -> ()  [unwired: 2 in, 2 out]
  n72 = Concatenate Strings(w60, "];" ("string")) -> (w43:string)
  n73 = Concatenate Strings(w45, "];" ("string 7")) -> (w38:string)
  n74 = Concatenate Strings(w47, "];" ("string 5")) -> (w40:string)
  n75 = Concatenate Strings(w48, "];" ("string 4")) -> (w41:string)
  n76 = Concatenate Strings(w46, "];" ("string 6")) -> (w39:string)
  n77 = Concatenate Strings(w2, "];" ("string 2")) -> (w42:string)
  n78 = Concatenate Strings(w43, w42, w41, w40, w39, w38) -> (w1:string)
  n79 = case shown="No Error" w31 {
    selector: w31 -> [w191 _]
    tunnel: w3 -> [w194 _]
    tunnel: 0 ("offset (0)") -> [w193 _]
    tunnel: 2 ("length (rest)") -> [w192 _]
    tunnel: w1 -> [w190 _]
    tunnel: w1 -> [w188 _]
    frame No Error {
      # "Decide if\nwe want to\ncreate a pdf"
      n80 = case shown="True" "Create PDF" {
        tunnel: w194 -> [_ w229]
        tunnel: w193 -> [_ w228]
        tunnel: w192 -> [_ w227]
        tunnel: w191 -> [_ w210]
        tunnel: w190 -> [_ w211]
        tunnel: w188 -> [_ w206]
        frame False {
        }
        frame True {
          # "Write the main.m file"
          # "Write the Vectors into a .m file"
          # "Write the string for the main.m file \nfor the matlabcaller and decide the band colours"
          n81 = Current VI's Path() -> (path=w217:path)
          n82 = String Subset(string=w229, offset (0)=w228, length (rest)=w227) -> (substring=w202:string)
          n83 = call "Matlab String(SubVI).vi"("name"=w202, "band touch win"="band touch win", "band touch loose"="band touch loose") -> ("String"=w218:string)  [unwired: 8 in]
          "concatenated string" <- w218
          n84 = Strip Path(path=w217) -> (stripped path=w216:path)  [unwired: 1 out]
          "stripped path txt file 3" <- w216
          n85 = Build Path(base path=w216, name or relative path="Tlist.m") -> (appended path=w214:path)
          n86 = Open/Create/Replace File(file path (use dialog)=w214, error in=w210, operation (0:open)=T6."replace or create" ("operation (0:open) 2")) -> (refnum out=w213:refnum<file>, error out=w209:errorcluster)  [unwired: 3 in, 1 out]
          n87 = Write to Text File(file (use dialog)=w213, text=w211, error in=w209) -> (refnum out=w212:refnum<file>, error out=w199:errorcluster)  [unwired: 1 in, 1 out]
          n88 = Current VI's Path() -> (path=w226:path)
          n89 = Strip Path(path=w226) -> (stripped path=w225:path)  [unwired: 1 out]
          "stripped path txt file 2" <- w225
          n90 = Close File(refnum=w212, error in=w199) -> (error out=w198:errorcluster)  [unwired: 1 out]
          n91 = Concatenate Strings("Analyse", w202, ".m" ("string")) -> (w200:string)
          n92 = Build Path(base path=w225, name or relative path=w200) -> (appended path=w219:path)
          n93 = Open/Create/Replace File(file path (use dialog)=w219, error in=w198, operation (0:open)=T6."replace or create") -> (refnum out=w233:refnum<file>, error out=w230:errorcluster)  [unwired: 3 in, 1 out]
          n94 = Write to Text File(file (use dialog)=w233, text=w218, error in=w230) -> (refnum out=w232:refnum<file>, error out=w197:errorcluster)  [unwired: 1 in, 1 out]
          "error out 2" <- w197
          n95 = Close File(refnum=w232, error in=w197) -> (error out=w196:errorcluster)  [unwired: 1 out]
          n96 = call "MP_LaunchMatlabScript4.vi"("error in (no error)"=w196, "matlab script path"=w219) -> ("error out"=w195:errorcluster, "standard output"=→"computed command line":string)  [unwired: 4 in, 4 out]
          n97 = case shown="True" "Open pdf" {
            tunnel: [w259 w265] -> w204
            tunnel: w195 -> [w259 w264]
            tunnel: w202 -> [_ w262]
            frame False {
            }
            frame True {
              # "Open the pdf"
              n98 = Current VI's Path() -> (path=w271:path)
              n99 = Strip Path(path=w271) -> (stripped path=w270:path)  [unwired: 1 out]
              n100 = Concatenate Strings("ScoreSheet", w262) -> (w260:string)
              n101 = Build Path(base path=w270, name or relative path=w260) -> (appended path=w269:path)
              n102 = Path To String(path=w269) -> (string=w268:string)
              n103 = Format Into String(format string="open '%s.pdf'", error in=w264, w268) -> (resulting string=w266:string, error out=w263:errorcluster)  [unwired: 1 in]
              n104 = call <vilib>:"System Exec.vi"("wait until completion? (T)"=FALSE, "error in (no error)"=w263, "command line"=w266) -> ("error out"=w265:errorcluster)  [unwired: 5 in, 3 out]
            }
          }
          n105 = case shown="No Error" w204 {
            selector: w204 -> [w234 w258]
            tunnel: "Open Scoresheet" -> [w238 _]
            tunnel: w202 -> [w237 _]
            tunnel: [w236 w256] -> w207
            tunnel: [w235 w257] -> w205
            frame No Error {
              n106 = case shown="True" w238 {
                tunnel: w237 -> [_ w243]
                tunnel: w234 -> [w240 w249]
                tunnel: [w240 w246] -> w235
                tunnel: ["" ("String 2") w241] -> w236
                frame False {
                }
                frame True {
                  # "Read out the content of Summary"
                  n107 = Current VI's Path() -> (path=w255:path)
                  n108 = Strip Path(path=w255) -> (stripped path=w254:path)  [unwired: 1 out]
                  n109 = Concatenate Strings("Summary", w243, ".txt" ("string")) -> (w252:string)
                  n110 = Build Path(base path=w254, name or relative path=w252) -> (appended path=w244:path)
                  n111 = Open/Create/Replace File(file path (use dialog)=w244, error in=w249) -> (refnum out=w250:refnum<file>, error out=w248:errorcluster)  [unwired: 4 in, 1 out]
                  n112 = Read from Text File(file (use dialog)=w250, count="Count Summary", error in=w248) -> (refnum out=w251:refnum<file>, text=w241:string, error out=w247:errorcluster)  [unwired: 1 in, 1 out]
                  n113 = Close File(refnum=w251, error in=w247) -> (error out=w246:errorcluster)  [unwired: 1 out]
                  "String" <- w243
                }
              }
            }
            frame Error {
              n114 = call <vilib>:"Simple Error Handler.vi"("error in (no error)"=w258) -> ("error out"=w257:errorcluster, "message"=w256:string)  [unwired: 4 in, 3 out]
            }
          }
          "Summary output" <- w207
          "error out" <- w205
          "T list string" <- w206
        }
      }
    }
    frame Error {
    }
  }
